vi "configure.vi"(8 "error in (no error)":errorcluster, 9 "Value":i32, 10 "ILC":refnum<class "ILC.lvclass">, 11 "ConfigureILCMotorDriveStrategy in":refnum<class "ConfigureILCMotorDriveStrategy.lvclass">) -> (0 "error out":errorcluster, 2 "ILC 2":refnum<class "ILC.lvclass">, 3 "ConfigureILCMotorDriveStrategy out":refnum<class "ConfigureILCMotorDriveStrategy.lvclass">)   [LabVIEW 2016, in "ConfigureILCMotorDriveStrategy.lvclass"]
uses:
  ConfigureILCMotorDriveStrategy.lvclass
  Common_ILC/ILC/ILC.lvclass
  ConfigureILCMotorDriveStrategy.lvclass/ConfigureILCMotorDriveStrategy.ctl
  Common_ILC/ILC/ILC.lvclass/ILC.ctl
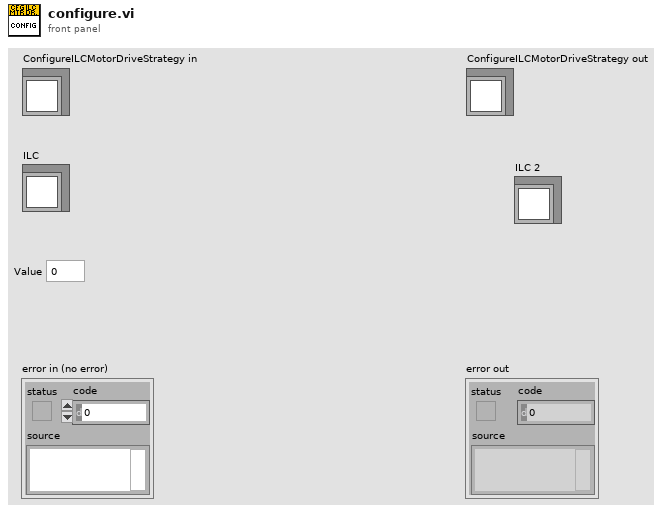
[diagram p1: front panel]
types:
  T1 = typedef "ILCBTTypedefs.lvlib/MUX Signals.ctl" = cluster{"MUX_A0 DAQ Channel to Write":refnum<k21>, "MUX_A1 DAQ Channel to Write":refnum<k21>}
  T2 = typedef "ILCBTTypedefs.lvlib/MUX Settings.ctl" = cluster{"MUX_AO":T3, "MUX_A1":T3}
  T3 = typedef "ILCBTTypedefs.lvlib/Digital Signal Level.ctl" = enum16{"Low", "High"}
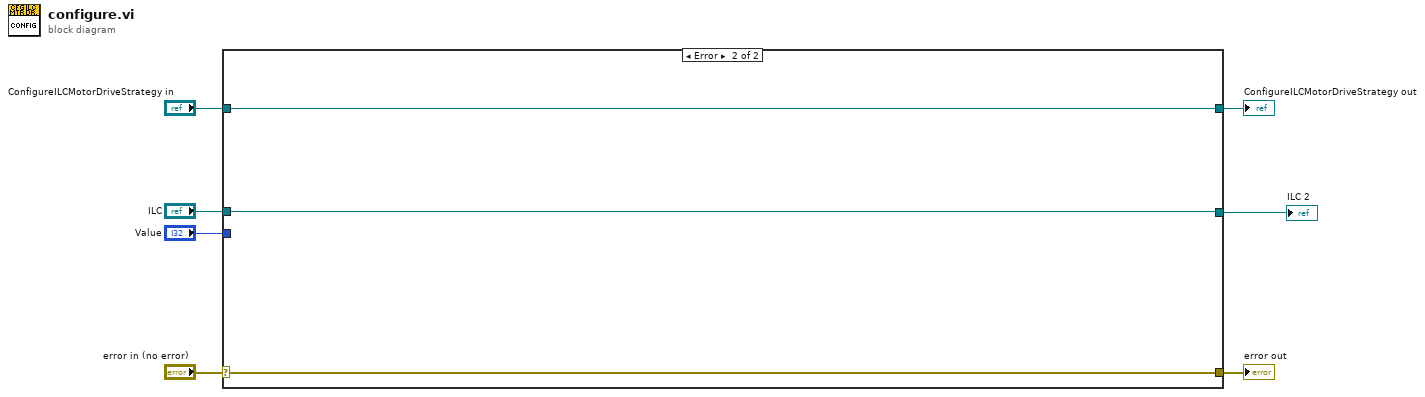
[diagram p0: block diagram]
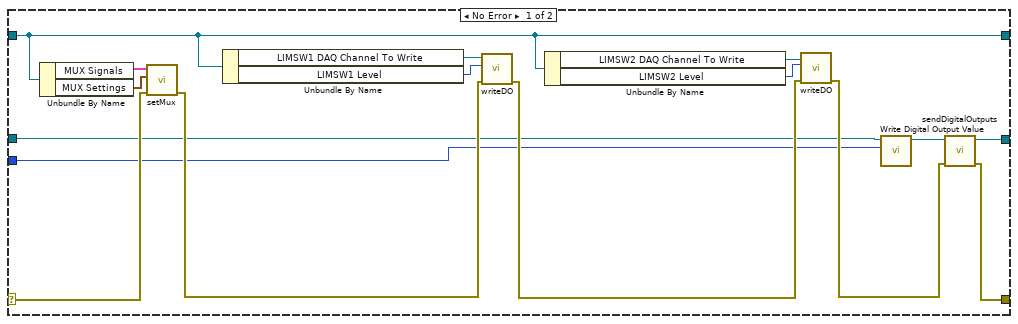
[diagram p2: hidden frame]
diagram:
  n1 = case shown="Error" "error in (no error)" {
    selector: "error in (no error)" -> [w22 w26]
    tunnel: [w21 w26] -> w6
    tunnel: [w19 w25] -> w4
    tunnel: "ConfigureILCMotorDriveStrategy in" -> [w19 w25]
    tunnel: "ILC" -> [w10 w24]
    tunnel: "Value" -> [w9 _]
    tunnel: [w8 w24] -> w1
    frame No Error {
      n2 = Unbundle By Name(w19) -> ("MUX Signals"=w23:T1, "MUX Settings"=w12:T2)
      n3 = call "setMux.vi"("error in (no error)"=w22, "MUX Settings"=w12, "MUX Signals"=w23) -> ("error out"=w13:errorcluster)  [unwired: 8 in]
      n4 = Unbundle By Name(w19) -> ("LIMSW1 DAQ Channel To Write"=w18:refnum<k21>, "LIMSW1 Level"=w20:T3)
      n5 = call "writeDO.vi"("error in"=w13, "Digital Signal Level"=w20, "DAQmx Global Channel"=w18) -> ("error out"=w15:errorcluster)  [unwired: 8 in]
      n6 = Unbundle By Name(w19) -> ("LIMSW2 DAQ Channel To Write"=w17:refnum<k21>, "LIMSW2 Level"=w16:T3)
      n7 = call "writeDO.vi"("error in"=w15, "Digital Signal Level"=w16, "DAQmx Global Channel"=w17) -> ("error out"=w14:errorcluster)  [unwired: 8 in]
      n8 = call "Write Digital Output Value.vi"("Digital Output Value"=w9, "ILC in"=w10) -> ("ILC out"=w11:refnum<class "ILC.lvclass">)  [unwired: 9 in]
      n9 = call "sendDigitalOutputs.vi"("error in (no error)"=w14, "ILC in"=w11) -> ("error out"=w21:errorcluster, "ILC out"=w8:refnum<class "ILC.lvclass">)  [unwired: 8 in]
    }
    frame Error {
    }
  }
  "error out" <- w6
  "ConfigureILCMotorDriveStrategy out" <- w4
  "ILC 2" <- w1
